vi "getSumsDSK.vi"(11 "Tabel as Arr":string[](array[string])) -> (3 "Sum as DBL":dbl[](array[numeric]))   [LabVIEW 2023]
panel:
  out "Sum as Str":string[](array[string])
  out "before 1 sub":string
  out "before 2 sub":string
  out "concatenated string":string
  out "double precision float":dbl format="%#_8g"
  in  "default (0 I32)":u32
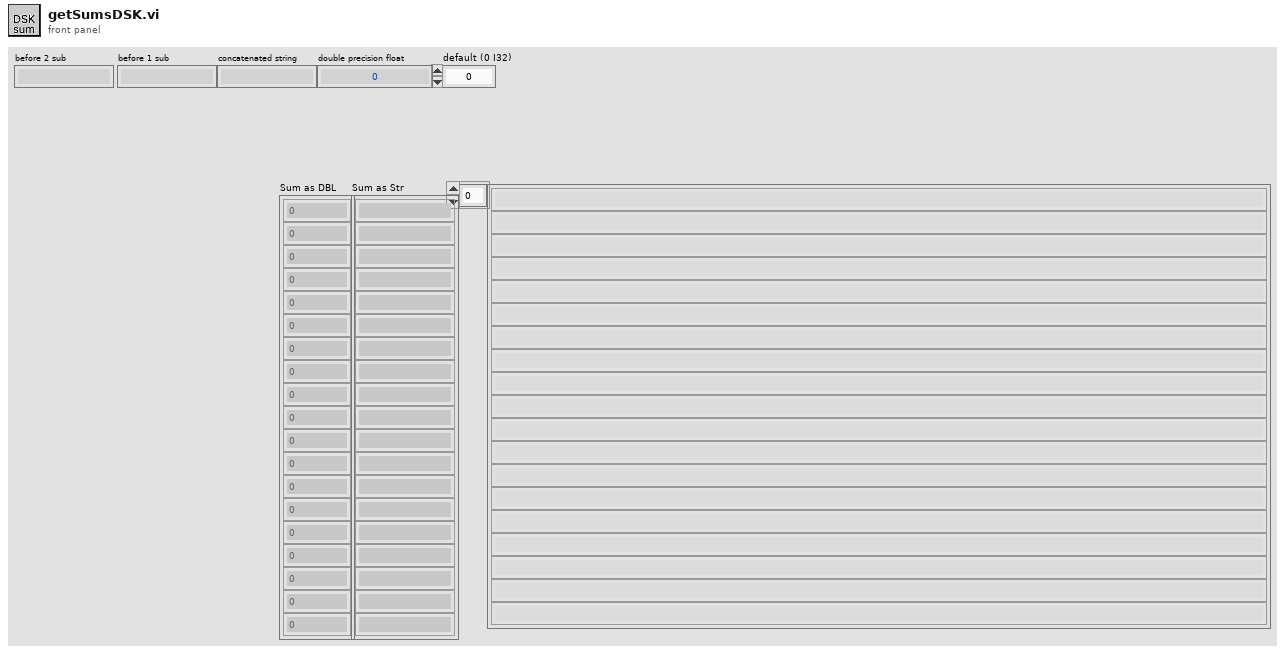
[diagram p1: front panel]
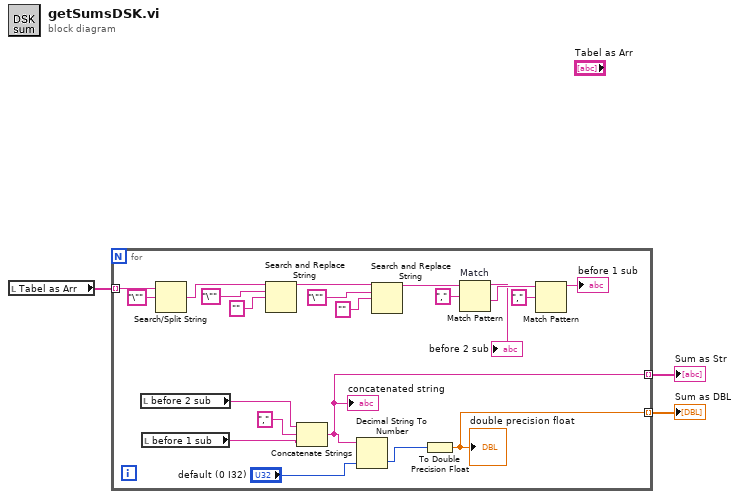
[diagram p0: block diagram]
diagram:
  n1 = local read "Tabel as Arr"() -> (w3:string[])
  n2 = for {
    tunnel: w3 -> [w24] mode=indexing
    tunnel: [w7] -> w2 mode=indexing
    tunnel: [w4] -> w1 mode=indexing
    n3 = local read "before 2 sub"() -> (w8:string)
    n4 = local read "before 1 sub"() -> (w10:string)
    n5 = Search/Split String(string=w24, search string/char (-)="\"") -> (match + rest of string=w22:string)  [unwired: 1 in, 2 out]
    n6 = Search and Replace String(input string=w22, search string="\"", replace string="" ("replace string (\"\")")) -> (result string=w17:string)  [unwired: 5 in, 3 out]
    n7 = Concatenate Strings "Concatenate Strings"(w8, ",", w10) -> (w7:string)
    "concatenated string" <- w7
    n8 = Decimal String To Number(string=w7, default (0L)="default (0 I32)") -> (number=w6:u32)  [unwired: 1 in, 1 out]
    n9 = Search and Replace String(input string=w17, search string="\"", replace string="" ("replace string (\"\")")) -> (result string=w12:string)  [unwired: 5 in, 3 out]
    n10 = To Double Precision Float(number=w6) -> (double precision float=w4:dbl)
    "double precision float" <- w4
    n11 = Match Pattern "Match"(string=w12, regular expression=",") -> (before substring=→"before 2 sub":string, after substring=w14:string)  [unwired: 1 in, 2 out]
    n12 = Match Pattern(string=w14, regular expression=",") -> (before substring=→"before 1 sub":string)  [unwired: 1 in, 3 out]
  }
  "Sum as Str" <- w2
  "Sum as DBL" <- w1
